vi "Ascii string to Hex string.vi"(1 "ASCII String":string) -> (0 "HEX String":string)   [LabVIEW 2016]
doc: "Converts normal string to hex string\n\n\nby: ian f koo\nemail: labview@ianfung.net\ndate: 08/2003"
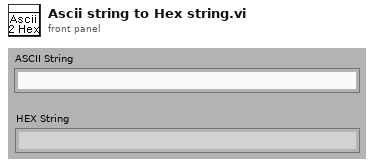
[diagram p1: front panel]
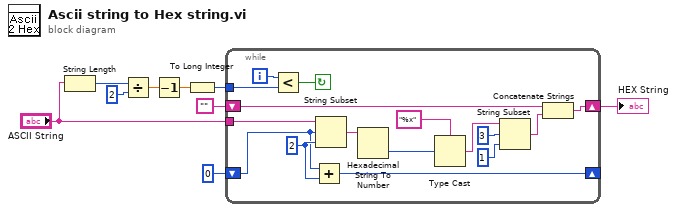
[diagram p0: block diagram]
diagram:
  n1 = String Length(string="ASCII String") -> (length=w8:i32)
  n2 = Divide(x=w8, y=2) -> (x/y=w6:dbl)
  n3 = Decrement(x=w6) -> (x-1=w4:dbl)
  n4 = To Long Integer(number=w4) -> (32bit integer=w3:i32)
  n5 = while {
    tunnel: "ASCII String" -> [w25]
    tunnel: w3 -> [w20]
    shift-right: [w16] -> _
    shift-left: 0 ("length (rest)") -> [w15]
    shift-right: [w13] -> w1
    shift-left: "" -> [w14]
    i -> [w17]
    stop <- w19 continue-if-true
    w18 = 2 ("length (rest)")
    n6 = Less?(x=w17, y=w20) -> (x < y?=w19:bool)
    n7 = Add(x=w15, y=w18) -> (x+y=w16:i32)
    n8 = String Subset(string=w25, offset (0)=w15, length (rest)=w18) -> (substring=w23:string)
    n9 = Hexadecimal String To Number(string=w23) -> (number=w24:u32)  [unwired: 2 in, 1 out]
    n10 = Type Cast(type="%x", x=w24) -> (*(type *) &x=w22:string)
    n11 = String Subset(string=w22, offset (0)=3, length (rest)=1 ("length (rest)")) -> (substring=w21:string)
    n12 = Concatenate Strings(w14, w21) -> (w13:string)
  }
  "HEX String" <- w1
